vi "Set-control-string.vi"(8 "error in (no error)":errorcluster, 9 "Value":string, 10 "Control name":T1, 11 "Panes in":T2) -> (0 "error out":errorcluster, 3 "Panes out":T2)   [LabVIEW 2013, in "MaterialCharacterization.lvlib" / "MC-UI.lvclass"]
uses:
  MC-UI.lvclass
  Panes-reference.ctl
  Control-names.ctl
  MC-UI.lvclass/MC-UI.ctl
  Read Controls lib.vi
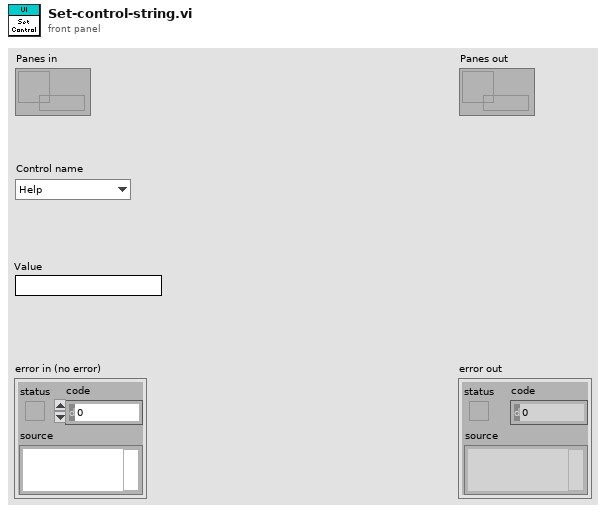
[diagram p1: front panel]
types:
  T1 = typedef "MaterialCharacterization.lvlib/MC-UI.lvclass/Control-names.ctl" = enum16{"Help", "Status", "Load configuration", "Save configuration", "Activate", "Start", "Stop", "Options"}
  T2 = typedef "MaterialCharacterization.lvlib/MC-UI.lvclass/Panes-reference.ctl" = refnum<data-value>
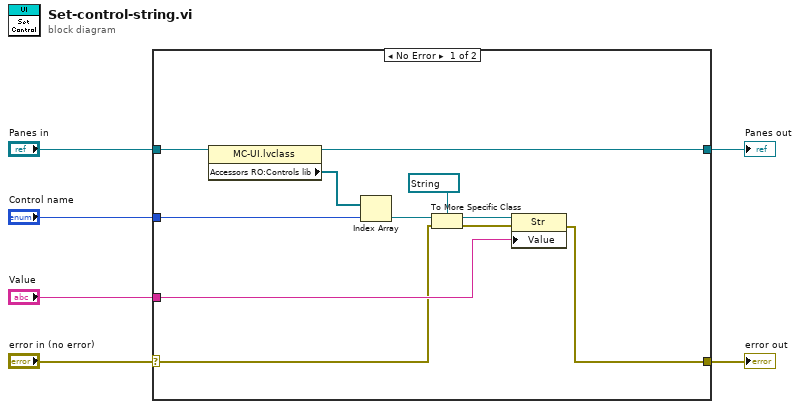
[diagram p0: block diagram]
diagram:
  n1 = case shown="No Error" "error in (no error)" {
    selector: "error in (no error)" -> [w9 w18]
    tunnel: [w12 w18] -> w5
    tunnel: [w11 w19] -> w3
    tunnel: "Panes in" -> [w17 w19]
    tunnel: "Control name" -> [w15 _]
    tunnel: "Value" -> [w13 _]
    frame No Error {
      n2 = property class="MC-UI.lvclass"(reference=w17) -> (reference out=w11:T2, "Accessors RO:Controls lib"=w16:refnum<vi>[])  [unwired: 1 in, 1 out]
      n3 = Index Array(array=w16, index=w15) -> (element=w14:refnum<vi>)
      n4 = To More Specific Class(target class=refnum<vi> refnum ("Value"), reference=w14, error in=w9) -> (specific class reference=w10:refnum<vi>, error out=w8:errorcluster)
      n5 = property class="Str"(reference=w10, error in=w8, "Value"=w13) -> (error out=w12:errorcluster)  [unwired: 1 out]
    }
    frame Error {
    }
  }
  "error out" <- w5
  "Panes out" <- w3
